vi "tearDown.vi"(8 "error in":errorcluster, 11 "reference in":refnum<class "SharedUtilities.lvclass">) -> (0 "error out":errorcluster, 3 "reference out":refnum<class "SharedUtilities.lvclass">)   [LabVIEW 2020, in "SharedUtilities.lvclass"]
doc: "tearDown runs after the test method has completed. Use this method to clean up any operations or references that were opened by setUp or the test method. Unit tests should be independent of other unit tests so this VI should ensure that the next test can run in a 'clean' test environment."
uses:
  SharedUtilities.lvclass
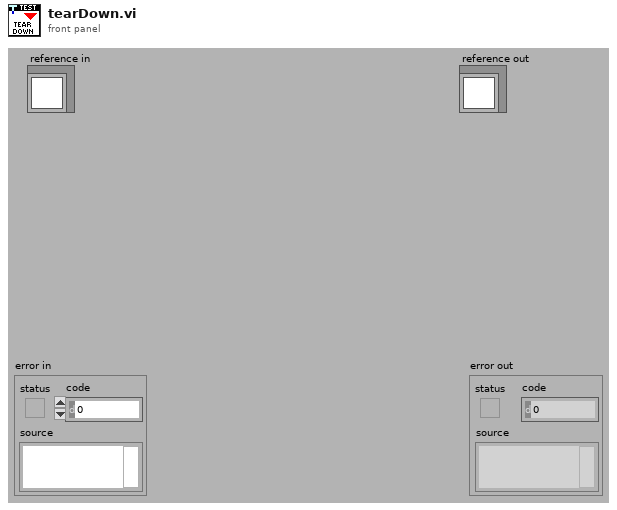
[diagram p1: front panel]
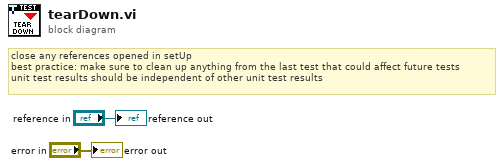
[diagram p0: block diagram]
diagram:
  # "close any references opened in setUp\nbest practice: make sure to clean up anything from the last test that could affect future tests\nunit test results should be independent of other unit test results"
  "error out" <- "error in"
  "reference out" <- "reference in"
